vi "rwr_Destroy gRPC Server.vi"(4 "Show in Debugger?":bool=TRUE, 6 "Message Priority":T1=enum."Normal", 7 "Caller in":refnum<class "Worker.lvclass">, 8 "error in":errorcluster, 9 "timeout (ms)":i32=5000, 10 "Data in":T3, 11 "gRPC Server in":refnum<class "gRPC Server.lvclass">) -> (0 "error out":errorcluster, 2 "Reply Data out":T2, 3 "dup gRPC Server out":refnum<class "gRPC Server.lvclass">, 5 "dup Caller out":refnum<class "Worker.lvclass">)   [LabVIEW 2019, in "gRPC Server (scope.proto).lvlib" / "gRPC Server.lvclass"]
doc: "This VI sends a <b>Public API Request with Reply</b> message to an MHL case of the Worker that owns this VI. This VI will wait until it receives a <b>Reply</b> message back from the Worker that owns this VI. If the wait time exceeds <b>timeout (ms)</b>, an error will be returned.\n---\nDestroys the bidi gRPC Server and closes al open connections"
uses:
  gRPC Server.lvclass
  <vilib>/addons/_Workers/Library/Classes/Worker/Worker.lvclass
  <vilib>/addons/_Workers/Library/Case Label.ctl
  <vilib>/addons/_Workers/Library/Workers.lvlib
  <vilib>/addons/_Workers/Library/Classes/Message/Priority.ctl
  <vilib>/addons/_Workers/Library/Classes/Message/Message.lvclass
  rwr_Destroy gRPC Server.ctl
  rwr_Destroy gRPC Server Reply.ctl
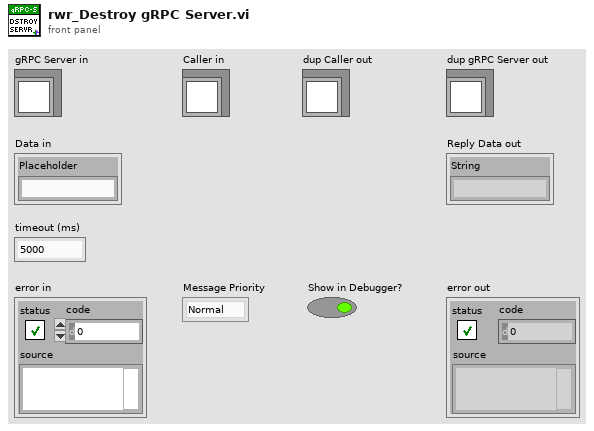
[diagram p1: front panel]
types:
  T1 = typedef "Workers.lvlib/Message.lvclass/Priority.ctl" = enum16{"Low", "Normal", "High"}
  T2 = typedef "gRPC Server (scope.proto).lvlib/gRPC Server.lvclass/rwr_Destroy gRPC Server Reply.ctl" = cluster{"String":string}
  T3 = typedef "gRPC Server (scope.proto).lvlib/gRPC Server.lvclass/rwr_Destroy gRPC Server.ctl" = cluster{"Placeholder":string}
  T4 = typedef "Workers.lvlib/Case Label.ctl" = string
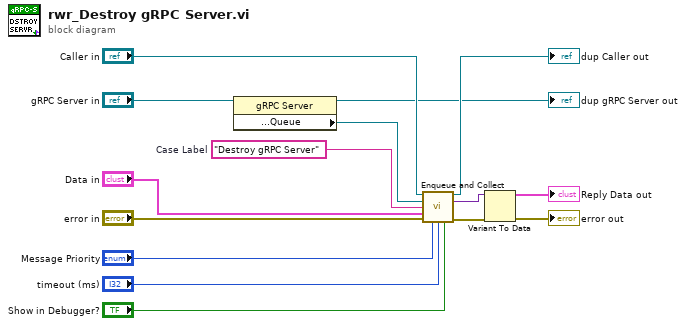
[diagram p0: block diagram]
diagram:
  w1 = T4 "Destroy gRPC Server"  # Case Label
  n1 = property class="gRPC Server"(reference="gRPC Server in") -> (reference out=→"dup gRPC Server out":refnum<class "gRPC Server.lvclass">, "Accessors:Read:Public API:Queue"=w2:refnum<class "Message Queue.lvclass">)  [unwired: 1 in, 1 out]
  n2 = call-dynamic "Enqueue and Collect.vi"("Worker"="Caller in", "Message Queue"=w2, "Case Label"=w1, "Data"="Data in", "error in (no error)"="error in", "Priority (Normal)"="Message Priority", "timeout in ms"="timeout (ms)", "Send Message to Debugger? (T)"="Show in Debugger?") -> ("dup Worker out"=→"dup Caller out":refnum<class "Worker.lvclass">, "Data out"=w7:variant, "error out"=w8:errorcluster)  [unwired: 4 in, 1 out]
  n3 = Variant To Data(error in=w8, Variant=w7) -> (data=→"Reply Data out":T2, error out=→"error out":errorcluster)  [unwired: 1 in]
